vi "Terminal-Modbus-WriteRegisters.vi"(8 "error in (no error)":errorcluster caption="错误输入（无错误）", 9 "ModbusNResRef":refnum<notifier>, 10 "ModbusNReqRef":refnum<notifier>, 11 "簇":T1) -> (0 "error out":errorcluster caption="错误输出")   [LabVIEW 2014]
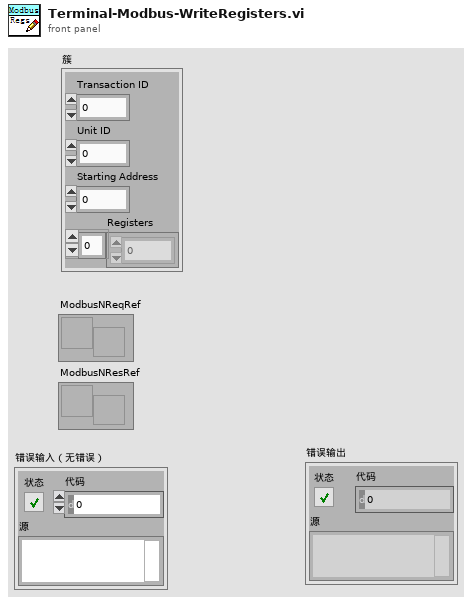
[diagram p1: front panel]
types:
  T1 = cluster{"Transaction ID":u16, "Unit ID":u8, "Starting Address":u16, "Registers":u16[]}
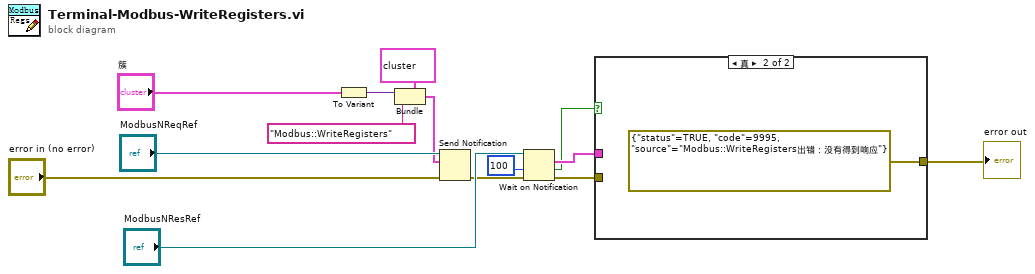
[diagram p0: block diagram]
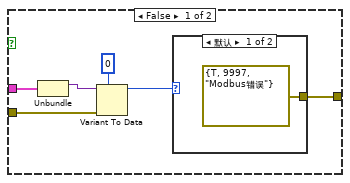
[diagram p2: hidden frame]
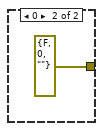
[diagram p3: hidden frame]
diagram:
  n1 = To Variant(anything="簇") -> (Variant=w12:variant)
  n2 = Bundle(cluster=cluster{variant, string} {variant, ""}, w12, "Modbus::WriteRegisters") -> (w10:cluster{variant, string})
  n3 = Send Notification(notification=w10, notifier="ModbusNReqRef", error in (no error)="error in (no error)") -> (error out=w9:errorcluster)  [unwired: 1 out]
  n4 = Wait on Notification(notifier="ModbusNResRef", timeout in ms (-1)=100 ("超时毫秒(-1)"), error in (no error)=w9) -> (notification=w7:cluster{variant, string}, timed out?=w2:bool, error out=w4:errorcluster)  [unwired: 1 in, 1 out]
  n5 = case shown="真" w2 {
    tunnel: w7 -> [w20 _]
    tunnel: w4 -> [w17 _]
    tunnel: [w15 errorcluster {"status"=TRUE, "code"=9995, "source"="Modbus::WriteRegisters出错：没有得到响应"} ("错误常量")] -> w3
    frame False {
      n6 = Unbundle(w20) -> (w19:variant)  [unwired: 1 out]
      n7 = Variant To Data(error in=w17, type=u8 0, Variant=w19) -> (data=w16:u8)  [unwired: 1 out]
      n8 = case shown="默认" w16 {
        tunnel: [errorcluster {"status"=TRUE, "code"=9997, "source"="Modbus错误"} ("错误常量") errorcluster {"status"=FALSE, "code"=0, "source"=""} ("错误常量")] -> w15
        frame Default {
        }
        frame 0 {
        }
      }
    }
    frame True {
    }
  }
  "error out" <- w3
